vi "Constructor.vi"(8 "error in (no error)":errorcluster, 10 "Connection Info":T1) -> (0 "error out":errorcluster, 3 "Postgres Connector Out":refnum<class "Postgres Connector.lvclass">)   [LabVIEW 2020, in "Postgres Connector.lvclass"]
doc: "VI used to enter the parameters before using the rest of the driver. \n\n*Important to use at the beginning of the code*"
uses:
  Postgres Connector.lvclass
  Postgres Connector.lvclass/Postgres Connector.ctl
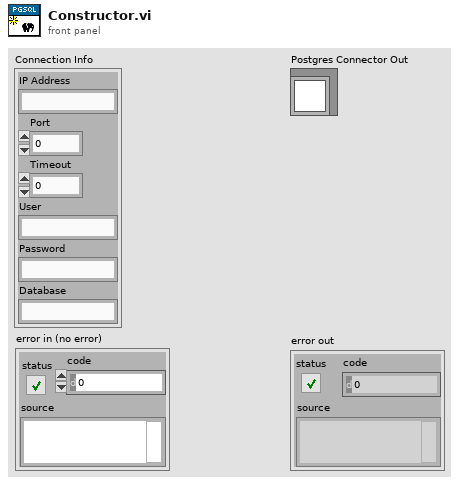
[diagram p1: front panel]
types:
  T1 = cluster{"IP Address":string, "Port":u16, "Timeout":i32, "User":string, "Password":string, "Database":string}
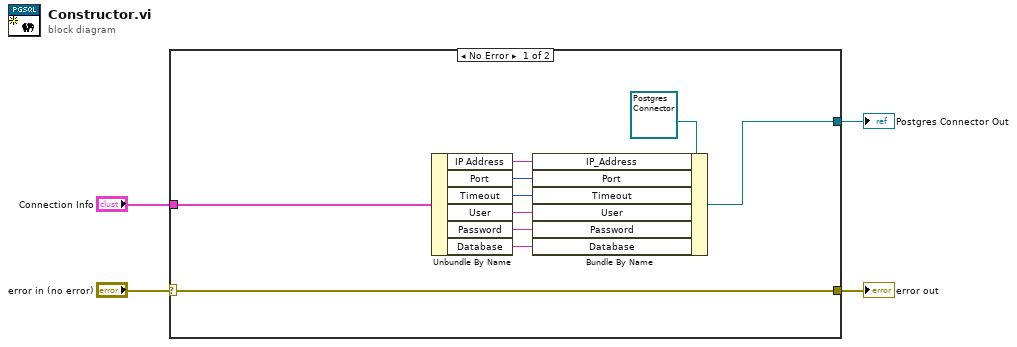
[diagram p0: block diagram]
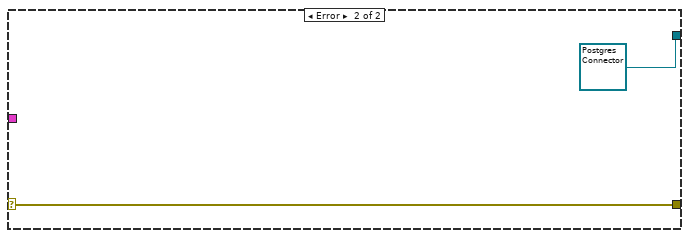
[diagram p2: hidden frame]
diagram:
  n1 = case shown="No Error" "error in (no error)" {
    selector: "error in (no error)" -> [w5 w16]
    tunnel: [w5 w16] -> w3
    tunnel: [w13 refnum<class "Postgres Connector.lvclass"> refnum ("Postgres Connector In")] -> w2
    tunnel: "Connection Info" -> [w14 _]
    frame No Error {
      n2 = Unbundle By Name(w14) -> ("IP Address"=w12:string, "Port"=w11:u16, "Timeout"=w10:i32, "User"=w9:string, "Password"=w8:string, "Database"=w6:string)
      n3 = Bundle By Name(cluster=refnum<class "Postgres Connector.lvclass"> refnum ("Postgres Connector In"), "IP_Address"=w12, "Port"=w11, "Timeout"=w10, "User"=w9, "Password"=w8, "Database"=w6) -> (w13:refnum<class "Postgres Connector.lvclass">)
    }
    frame Error {
    }
  }
  "Postgres Connector Out" <- w2
  "error out" <- w3
